vi "MTS_SaveImagePng.vi"(5 "Save .png":bool=TRUE, 6 "Tree Refnum":refnum<vi>, 7 ".pt3 File Name":path, 8 "error in":errorcluster, 11 "Image":i32[][](array[numeric])) -> (0 "error out":errorcluster)   [LabVIEW 2013]
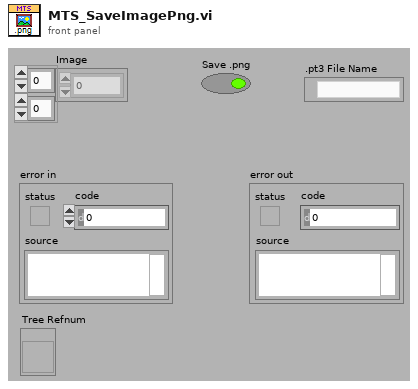
[diagram p1: front panel]
types:
  T1 = enum16{"unknown", "pt3 File", "png Image", "bmp Image"}
  T2 = enum16{"not a pt3 File", "Image File", "Point Measurement", "Auto Point"}
  T3 = typedef "Image Type" = u32
  T4 = typedef "IMAQ Image.ctl" = refnum<image>
  T5 = cluster{"File No":i32, "File Path":path, "Parent File":i32, "File Type":enum16{"unknown", "pt3 File", "png Image", "bmp Image"}, "Measurement Type":enum16{"not a pt3 File", "Image File", "Point Measurement", "Auto Point", "Line Scan", "Grid Scan"}, "Upper Left":cluster{"x-Position":dbl, "y-Position":dbl, "z-Position":dbl}, "Pixels":i32[], "Picture Size":dbl[], "Scan Axis":enum32{"x-y", "x-z", "y-z"}}
  T6 = cluster{"x-Position":dbl, "y-Position":dbl, "z-Position":dbl}
  T7 = cluster{"Picture Size":dbl[], "Pixels":i32[], "Upper Left":cluster{"x-Position":dbl, "y-Position":dbl, "z-Position":dbl}}
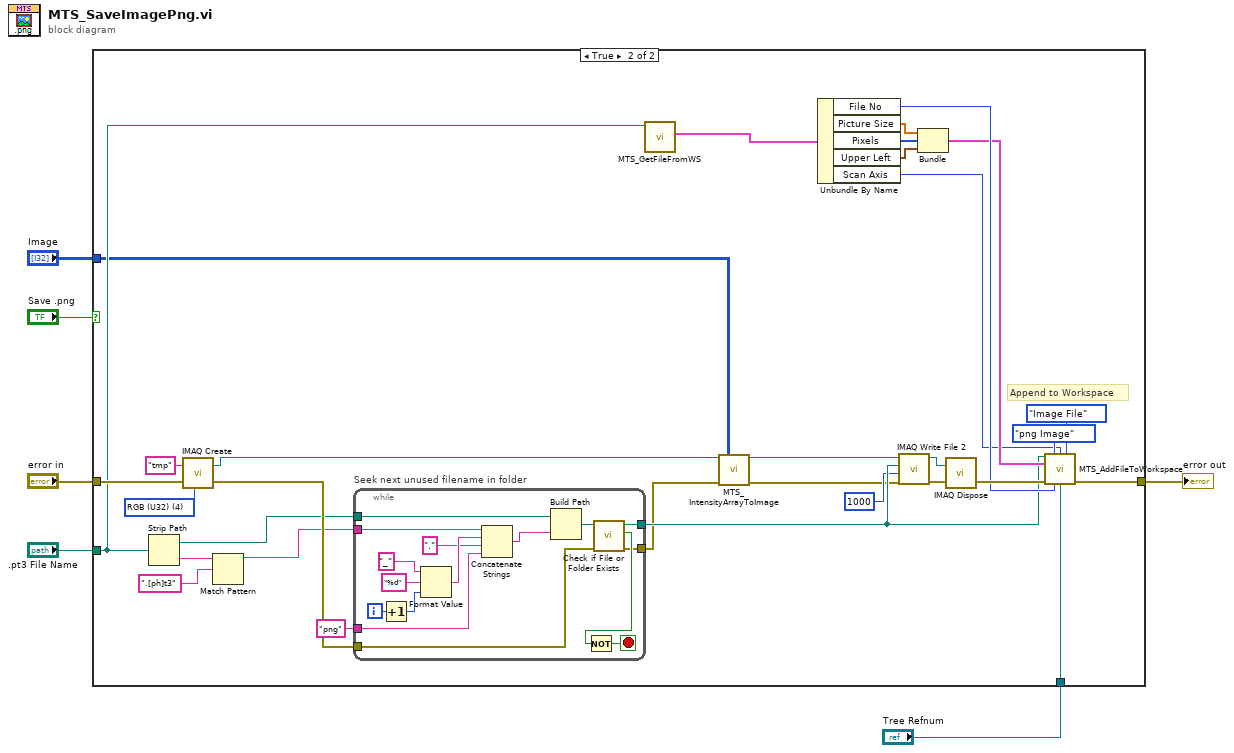
[diagram p0: block diagram]
diagram:
  n1 = case shown="True" "Save .png" {
    tunnel: "Image" -> [_ w9]
    tunnel: "error in" -> [w7 w38]
    tunnel: [w7 w27] -> w3
    tunnel: ".pt3 File Name" -> [_ w15]
    tunnel: "Tree Refnum" -> [_ w26]
    frame False {
    }
    frame True {
      w36 = T3 4 items=["Grayscale (U8)", "Grayscale (I16)", "Grayscale (SGL)", "Complex (CSG)", "RGB (U32)", "HSL (U32)", "RGB (U64)", "Grayscale (U16)"] ("Image Type")
      # "Append to Workspace"
      n2 = Strip Path(path=w15) -> (stripped path=w30:path, name=w33:string)
      n3 = call "IMAQ Create"("Image Name"="tmp", "Image Type"=w36, "error in (no error)"=w38) -> ("New Image"=w10:T4, "error out"=w31:errorcluster)  [unwired: 2 in]
      n4 = Match Pattern(string=w33, regular expression=".[ph]t3") -> (before substring=w8:string)  [unwired: 1 in, 3 out]
      n5 = while "Seek next unused filename in folder" {
        tunnel: w30 -> [w54]
        tunnel: [w49] -> w19
        tunnel: w31 -> [w48]
        tunnel: [w47] -> w13
        tunnel: w8 -> [w42]
        tunnel: "png" ("File Type") -> [w39]
        i -> [w44]
        stop <- w51 stop-if-true
        n6 = Increment(x=w44) -> (x+1=w43:i32)
        n7 = Format Value(string ("")="_", format string="%d", value (0)=w43) -> (output string=w45:string)
        n8 = Concatenate Strings(w42, w45, "." ("string"), w39) -> (w53:string)
        n9 = Build Path(base path=w54, name or relative path=w53) -> (appended path=w52:path)
        n10 = call <vilib>:"Check if File or Folder Exists.vi"("error in (no error)"=w48, "path"=w52) -> ("error out"=w47:errorcluster, "file or folder exists?"=w50:bool, "dup path"=w49:path)  [unwired: 7 in]
        n11 = Not(x=w50) -> (.not. x?=w51:bool)
      }
      n12 = call "MTS_GetFileFromWS.vi"(".pt3 File Name"=w15) -> ("File Header"=w16:T5)  [unwired: 9 in, 1 out]
      n13 = call "MTS_IntensityArrayToImage.vi"(0:"Image"=w10, 1:"Image"=w9, "error in (no error)"=w13) -> ("Image Out"=w11:T4, "error out"=w12:errorcluster)  [unwired: 11 in]
      n14 = Unbundle By Name(w16) -> ("File No"=w21:i32, "Picture Size"=w24:dbl[], "Pixels"=w23:i32[], "Upper Left"=w22:T6, "Scan Axis"=w14:enum32{"x-y", "x-z", "y-z"})
      n15 = call-poly "IMAQ Write File 2"("error in (no error)"=w12, "Image Quality"=u32 1000, "File Path"=w19, "Image"=w11) -> ("error out"=w35:errorcluster, "Image Out (duplicate)"=w34:T4)  [unwired: 6 in]
      n16 = Bundle("Picture Size"=w24, "Pixels"=w23, "Upper Left"=w22) -> (w20:T7)  [unwired: 1 in]
      n17 = call "IMAQ Dispose"("Image"=w34, "error in (no error)"=w35) -> ("error out"=w28:errorcluster)  [unwired: 4 in]
      n18 = call "MTS_AddFileToWorkspace.vi"("File Name"=w19, "File Type"=T1."png Image", "Scan Axis"=w14, "Measurement Type"=T2."Image File", "File Info"=w20, "error in (no error)"=w28, "Parent"=w21, "Tree Refnum"=w26) -> ("error out"=w27:errorcluster)  [unwired: 5 in, 2 out]
    }
  }
  "error out" <- w3
